vi "mkAdjustROIPositions.vi"(9 "Corner-based bead pos":cluster{"X":i32, "Y":i32}[](array[cluster]), 10 "Camera settings":T1={"Gain [1-4]"=50.0, "Offset"=2, "Mode"=75, "ROIs"=[], "ROI Size"={"X"=0, "Y"=0}, "Number of buffers"=40, "Use hardware multiple-ROI?"=TRUE, "GenericCameraConfig"={"Framerate (Hz)"=60, "Exposure time (us)"=5000, "Image size"={"Width"=1280, "Height"=1024}, "Number of buffers"=30}}) -> (1 "Adjusted bead pos (out)":cluster{"X":i32, "Y":i32}[](array[cluster]))   [LabVIEW 2011]
uses:
  CameraConfig.ctl
  Main/Camera/GenericCameraConfigType.ctl
panel:
  in  "Sort ROIs?":bool
  # "us"
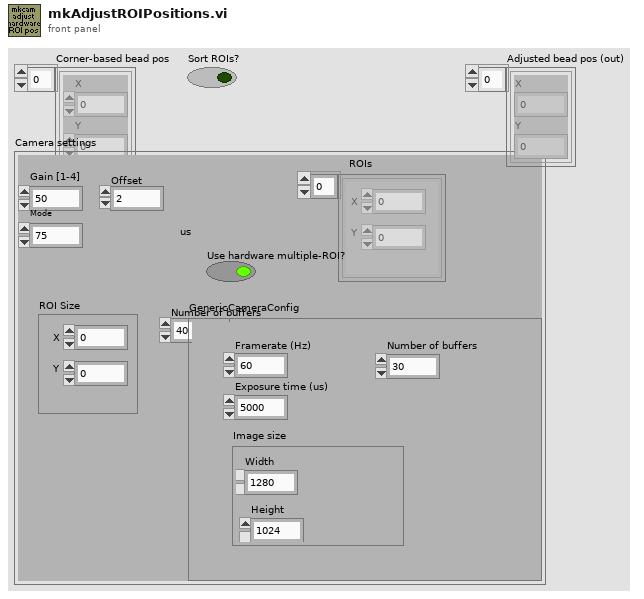
[diagram p1: front panel]
types:
  T1 = typedef "CameraConfig.ctl" = cluster{"Gain [1-4]":sgl, "Offset":i16, "Mode":i16, "ROIs":cluster{"X":i32, "Y":i32}[], "ROI Size":cluster{"X":i32, "Y":i32}, "Number of buffers":i32, "Use hardware multiple-ROI?":bool, "GenericCameraConfig":T2}
  T2 = typedef "GenericCameraConfigType.ctl" = cluster{"Framerate (Hz)":i32, "Exposure time (us)":i32, "Image size":cluster{"Width":i32, "Height":i32}, "Number of buffers":i32}
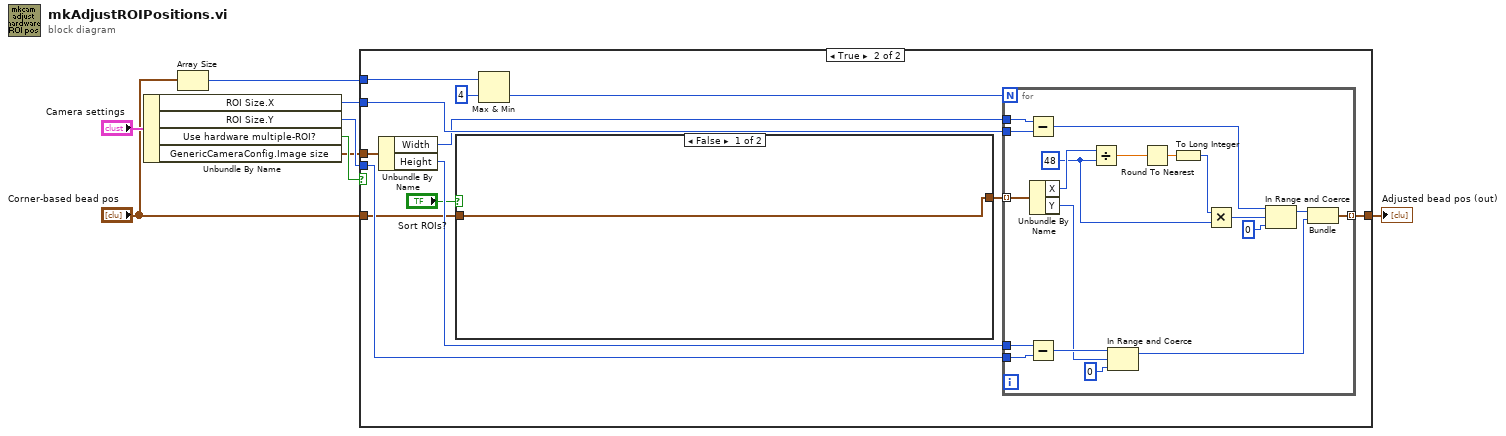
[diagram p0: block diagram]
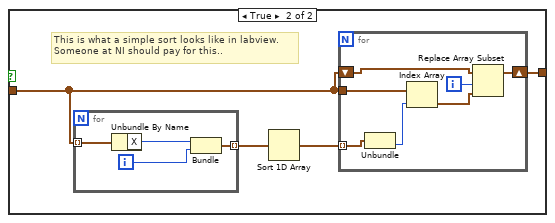
[diagram p3: hidden frame]
diagram:
  n1 = Unbundle By Name("Camera settings") -> ("ROI Size.X"=w7:i32, "ROI Size.Y"=w6:i32, "Use hardware multiple-ROI?"=w2:bool, "GenericCameraConfig.Image size"=w1:cluster{"Width":i32, "Height":i32})
  n2 = Array Size(array="Corner-based bead pos") -> (size(s)=w3:i32)
  n3 = case shown="True" w2 {
    tunnel: w7 -> [_ w21]
    tunnel: w6 -> [_ w20]
    tunnel: [w9 w19] -> w5
    tunnel: "Corner-based bead pos" -> [w9 w12]
    tunnel: w3 -> [_ w17]
    tunnel: w1 -> [_ w15]
    frame False {
    }
    frame True {
      n4 = Unbundle By Name(w15) -> ("Width"=w14:i32, "Height"=w13:i32)
      n5 = case shown="False" "Sort ROIs?" {
        tunnel: w12 -> [w22 w24]
        tunnel: [w22 w23] -> w11
        frame False {
        }
        frame True {
          # "This is what a simple sort looks like in labview.\nSomeone at NI should pay for this.."
          n6 = for {
            tunnel: w24 -> [w37] mode=indexing
            tunnel: [w34] -> w26 mode=indexing
            i -> [w35]
            n7 = Unbundle By Name(w37) -> ("X"=w36:i32)
            n8 = Bundle("X"=w36, w35) -> (w34:cluster{"X":i32, i32})  [unwired: 1 in]
          }
          n9 = Sort 1D Array(array=w26) -> (sorted array=w25:cluster{"X":i32, i32}[])
          n10 = for {
            tunnel: w25 -> [w29] mode=indexing
            tunnel: w24 -> [w32]
            shift-right: [w31] -> w23
            shift-left: w24 -> [w33]
            i -> [w27]
            n11 = Unbundle(w29) -> (w28:i32)  [unwired: 1 out]
            n12 = Index Array(array=w32, index=w28) -> (element=w30:cluster{"X":i32, "Y":i32})
            n13 = Replace Array Subset(array=w33, new element=w30, index=w27) -> (w31:cluster{"X":i32, "Y":i32}[])
          }
        }
      }
      n14 = Max & Min(x=w17, y=4) -> (min(x,y)=w16:i32)  [unwired: 1 out]
      n15 = for {
        N: w16 -> [_]
        tunnel: w11 -> [w56] mode=indexing
        tunnel: w21 -> [w48]
        tunnel: w20 -> [w46]
        tunnel: [w40] -> w19 mode=indexing
        tunnel: w14 -> [w39]
        tunnel: w13 -> [w38]
        w51 = 48 ("y")
        n16 = Subtract(x=w39, y=w48) -> (x-y=w47:i32)
        n17 = Subtract(x=w38, y=w46) -> (x-y=w45:i32)
        n18 = Unbundle By Name(w56) -> ("X"=w55:i32, "Y"=w44:i32)
        n19 = Divide(x=w55, y=w51) -> (x/y=w54:dbl)
        n20 = In Range and Coerce(upper limit=w45, x=w44, lower limit=0) -> (coerced(x)=w41:i32)  [unwired: 1 out]
        n21 = Round To Nearest(number=w54) -> (nearest integer value=w53:dbl)
        n22 = To Long Integer(number=w53) -> (32bit integer=w52:i32)
        n23 = Multiply(x=w52, y=w51) -> (x*y=w50:i32)
        n24 = In Range and Coerce(upper limit=w47, x=w50, lower limit=0) -> (coerced(x)=w42:i32)  [unwired: 1 out]
        n25 = Bundle("lower limit"=w42, "lower limit"=w41) -> (w40:cluster{"lower limit":i32, "lower limit":i32})  [unwired: 1 in]
      }
    }
  }
  "Adjusted bead pos (out)" <- w5
